vi "ReadWriteTest.vi"(8 "error in (no error)":errorcluster) -> (0 "error out":errorcluster)   [LabVIEW 2023, in "TestVIs.lvlib"]
uses:
  <vilib>/addons/_JKI Toolkits/Caraya/classes/Assert/Assert Equal Value_Variant.vi
  TestVIs.lvlib
  <vilib>/addons/_JKI Toolkits/Caraya/classes/Assert/Assert.lvclass
  <vilib>/addons/_JKI Toolkits/Caraya/classes/Test/Test.lvclass
  Library/Unit Testing CA1.lvlib
panel:
  # "READ WRITE TEST"
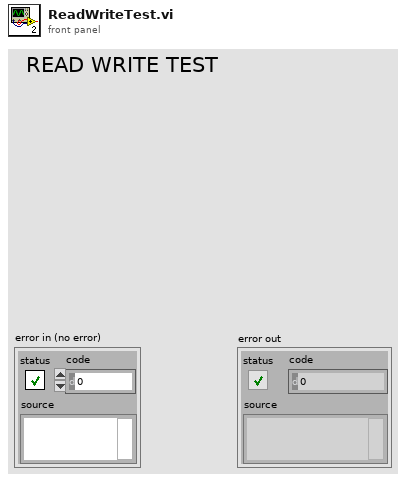
[diagram p1: front panel]
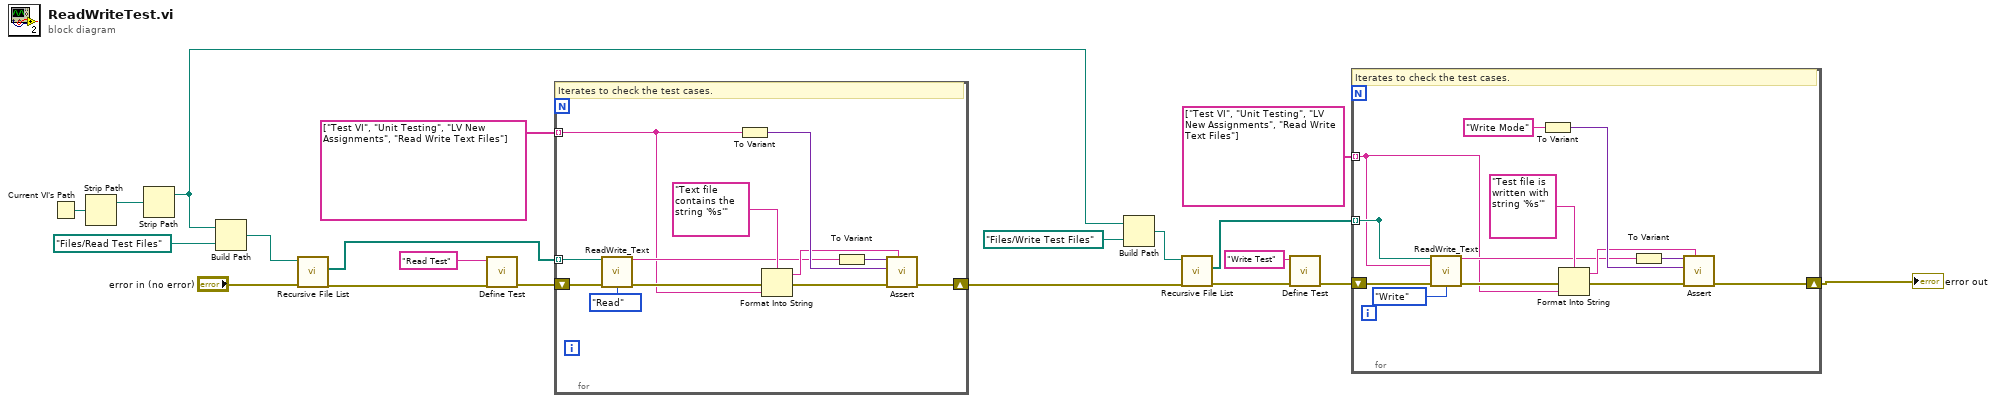
[diagram p0: block diagram]
diagram:
  n1 = Current VI's Path() -> (path=w20:path)
  n2 = Strip Path(path=w20) -> (stripped path=w16:path)  [unwired: 1 out]
  n3 = Strip Path(path=w16) -> (stripped path=w7:path)  [unwired: 1 out]
  n4 = Build Path(base path=w7, name or relative path=path "Files/Read Test Files") -> (appended path=w14:path)
  n5 = call <vilib>:"Recursive File List.vi"("error in (no error)"="error in (no error)", "Folder Path"=w14) -> ("error out"=w13:errorcluster, "All Files in Dir"=w11:path[])  [unwired: 5 in, 3 out]
  n6 = call <vilib>:"Define Test.vi"("error in (no error)"=w13, "Label (VI Title)"="Read Test") -> ("error out"=w17:errorcluster)  [unwired: 8 in, 1 out]
  n7 = for {
    tunnel: w11 -> [w25] mode=indexing
    shift-right: [w24] -> w6
    shift-left: w17 -> [w27]
    tunnel: string[] ["Test VI", "Unit Testing", "LV New Assignments", "Read Write Text Files"] ("Array") -> [w21] mode=indexing
    # "Iterates to check the test cases."
    n8 = call "ReadWrite_Text.vi"("file path"=w25, "error in"=w27, "Read/Write"=enum16{"Read", "Write"}."Read") -> ("Read String"=w23:string, "error out"=w26:errorcluster)  [unwired: 11 in]
    n9 = To Variant(anything=w21) -> (Variant=w32:variant)
    n10 = Format Into String(format string="Text file contains the string '%s'", error in=w26, w21) -> (resulting string=w28:string, error out=w30:errorcluster)  [unwired: 1 in]
    n11 = To Variant(anything=w23) -> (Variant=w31:variant)
    n12 = call-poly <vilib>:"Assert.vi"("Label"=w28, "error in (no error)"=w30, "Y"=w32, "X"=w31) -> ("error out"=w24:errorcluster)  [unwired: 6 in, 1 out]
  }
  n13 = Build Path(base path=w7, name or relative path=path "Files/Write Test Files") -> (appended path=w3:path)
  n14 = call <vilib>:"Recursive File List.vi"("error in (no error)"=w6, "Folder Path"=w3) -> ("error out"=w5:errorcluster, "All Files in Dir"=w4:path[])  [unwired: 5 in, 3 out]
  n15 = call <vilib>:"Define Test.vi"("error in (no error)"=w5, "Label (VI Title)"="Write Test") -> ("error out"=w9:errorcluster)  [unwired: 8 in, 1 out]
  n16 = for {
    tunnel: [w35] -> _ mode=indexing
    shift-right: [w38] -> w1
    shift-left: w9 -> [w40]
    tunnel: w4 -> [w35] mode=indexing
    tunnel: string[] ["Test VI", "Unit Testing", "LV New Assignments", "Read Write Text Files"] ("Array") -> [w33] mode=indexing
    # "Iterates to check the test cases."
    n17 = call "ReadWrite_Text.vi"("file path"=w35, "Write String"=w33, "error in"=w40, "Read/Write"=enum16{"Read", "Write"}."Write") -> ("Read String"=w37:string, "error out"=w39:errorcluster)  [unwired: 10 in]
    n18 = To Variant(anything="Write Mode" ("File/Folder Name")) -> (Variant=w45:variant)
    n19 = Format Into String(format string="Test file is written with string '%s'", error in=w39, w33) -> (resulting string=w41:string, error out=w43:errorcluster)  [unwired: 1 in]
    n20 = To Variant(anything=w37) -> (Variant=w44:variant)
    n21 = call-poly <vilib>:"Assert.vi"("Label"=w41, "error in (no error)"=w43, "Y"=w45, "X"=w44) -> ("error out"=w38:errorcluster)  [unwired: 6 in, 1 out]
  }
  "error out" <- w1
